vi "initial.vi"() -> (0 "monitor rsg handle":refnum<event-registration>, 1 "monitor interface":T1, 2 "event rsg handle":refnum<event-registration>, 3 "msg interface":T2, 4 "error out":errorcluster)   [LabVIEW 2013]
panel:
  out "新建？":bool
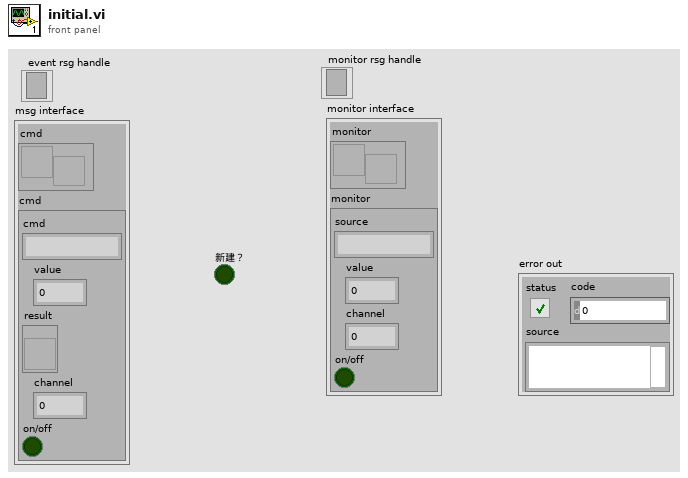
[diagram p1: front panel]
types:
  T1 = cluster{"monitor":refnum<user-event>, "monitor":cluster{"source":string, "value":dbl, "channel":i32, "on/off":bool}}
  T2 = cluster{"cmd":refnum<user-event>, "cmd":cluster{"cmd":string, "value":dbl, "result ":refnum<vi>, "channel":i32, "on/off":bool}}
  T3 = cluster{"source":string, "value":dbl, "channel":i32, "on/off":bool}
  T4 = cluster{"cmd":string, "value":dbl, "result ":refnum<vi>, "channel":i32, "on/off":bool}
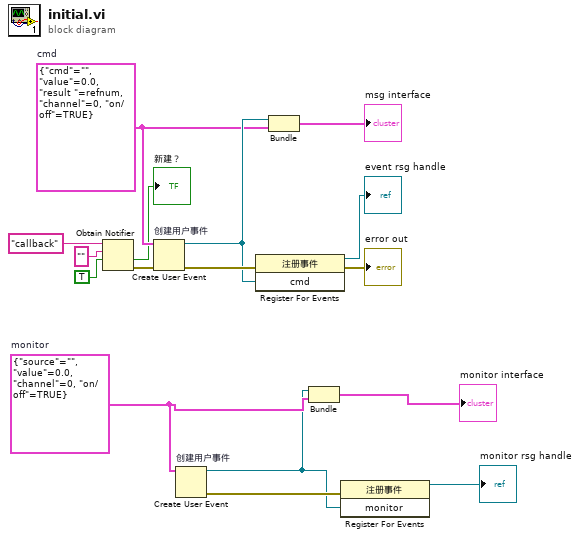
[diagram p0: block diagram]
diagram:
  w5 = T3 {"source"="", "value"=0.0, "channel"=0, "on/off"=TRUE}  # monitor
  w14 = T4 {"cmd"="", "value"=0.0, "result "=refnum, "channel"=0, "on/off"=TRUE}  # cmd
  n1 = Obtain Notifier(name (unnamed)="callback" ("名称（未命名）"), notification data type="", create if not found? (T)=TRUE ("如未找到是否创建？(T)")) -> (created new?=→"新建？":bool, error out=w6:errorcluster)  [unwired: 1 in, 1 out]
  n2 = Create User Event "创建用户事件"(user event datatype=w14, error in=w6) -> (user event=w15:refnum<user-event>, error out=w16:errorcluster)
  n3 = Create User Event "创建用户事件"(user event datatype=w5) -> (user event=w2:refnum<user-event>, error out=w3:errorcluster)  [unwired: 1 in]
  n4 = register-events(error in=w16, w15) -> (reference out=→"event rsg handle":refnum<event-registration>, error out=→"error out":errorcluster)  [unwired: 1 in]
  n5 = Bundle("cmd"=w15, "cmd"=w14) -> (→"msg interface":T2)  [unwired: 1 in]
  n6 = Bundle("monitor"=w2, "monitor"=w5) -> (→"monitor interface":T1)  [unwired: 1 in]
  n7 = register-events(error in=w3, w2) -> (reference out=→"monitor rsg handle":refnum<event-registration>)  [unwired: 1 in, 1 out]
